vi "Waveform_Execution2.vi"(2 "output cluster":T1) -> ()   [LabVIEW 2013]
uses:
  waveforms.ctl
  <vilib>/DAQmx/create/channels.llb/DAQmx Create Channel (AO-Voltage-Basic).vi
  <vilib>/DAQmx/create/channels.llb/DAQmx Create Channel (DO-Digital Output).vi
  <vilib>/Waveform/WDTOps.llb/WDT Number of Waveform Samples DBL.vi
  <vilib>/DAQmx/configure/timing.llb/DAQmx Timing (Sample Clock).vi
  <vilib>/DAQmx/write.llb/DAQmx Write (Analog 1D Wfm NChan NSamp).vi
  <vilib>/DAQmx/configure/trigger.llb/DAQmx Start Trigger (Digital Edge).vi
  <vilib>/DAQmx/write.llb/DAQmx Write (Digital 1D Wfm NChan NSamp).vi
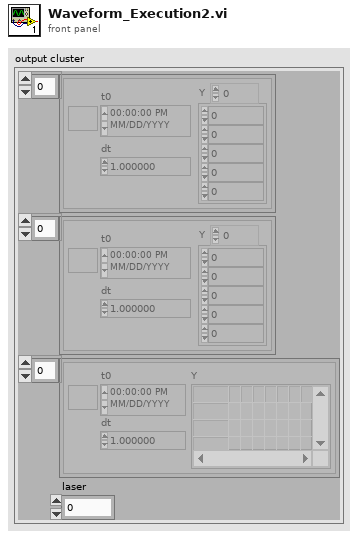
[diagram p1: front panel]
types:
  T1 = typedef "waveforms.ctl" = cluster{waveform(dbl)[], waveform(dbl)[], digitalwaveform[], "laser":i32}
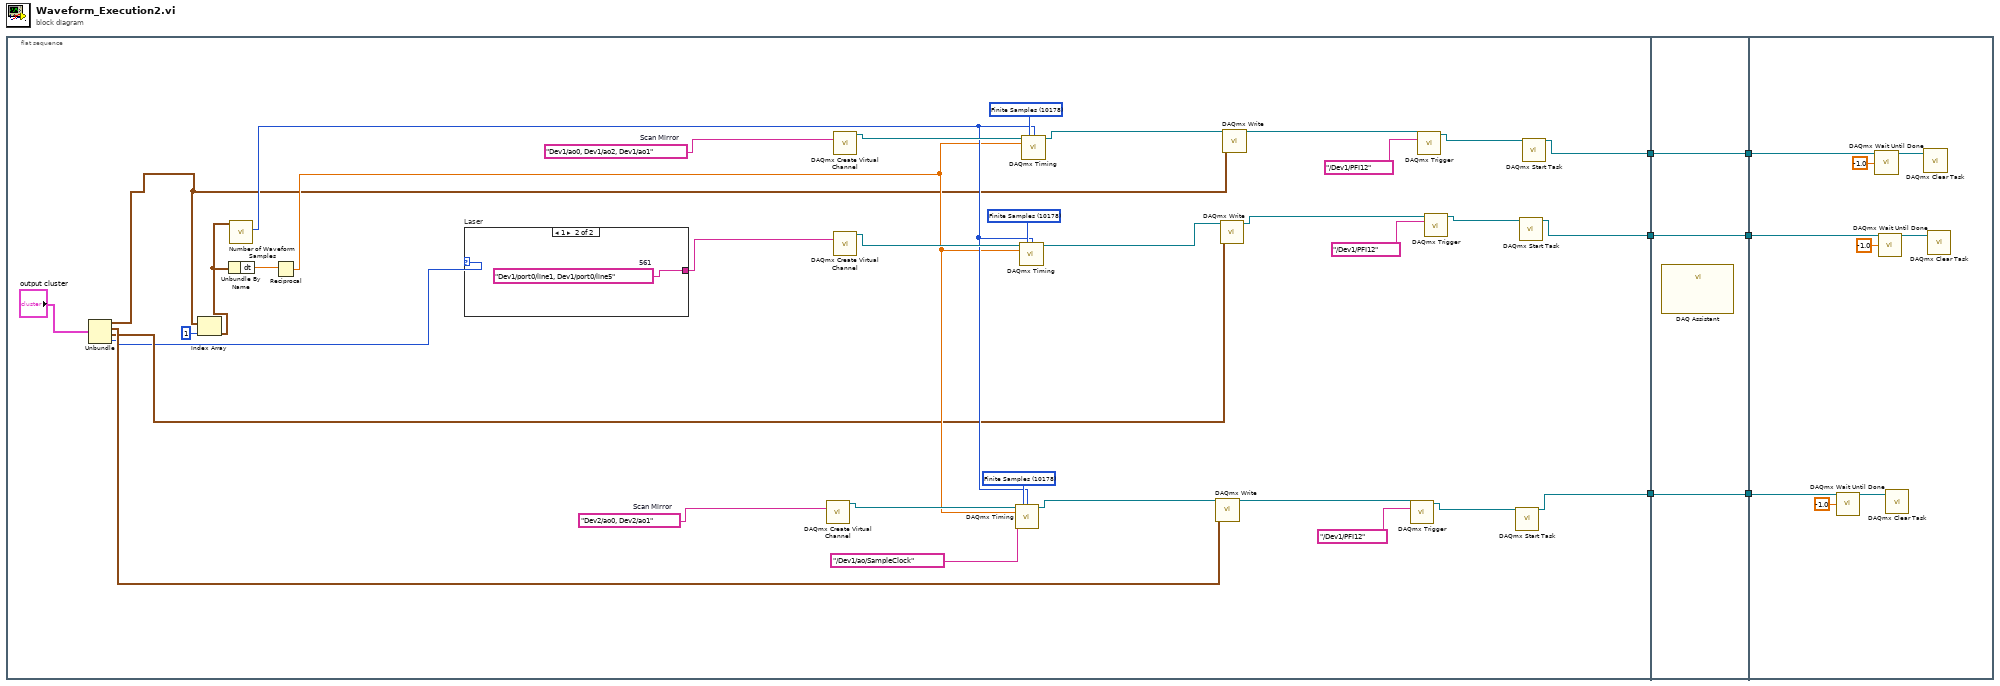
[diagram p0: block diagram]
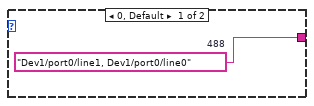
[diagram p2: hidden frame]
diagram:
  n1 = flat-sequence {
    tunnel: [w27] -> w5
    tunnel: [w26] -> w3
    tunnel: [w14] -> w1
    tunnel: [w46] -> w6
    tunnel: w5 -> [w46]
    tunnel: [w45] -> w4
    tunnel: w3 -> [w45]
    tunnel: [w44] -> w2
    tunnel: w1 -> [w44]
    tunnel: w6 -> [w53]
    tunnel: w4 -> [w52]
    tunnel: w2 -> [w47]
    frame #0 {
      w22 = 10178 items=["Finite Samples"=10178, "Continuous Samples"=10123, "Hardware Timed Single Point"=12522] ("sample mode")
      w23 = tag "Dev2/ao0, Dev2/ao1"  # Scan Mirror
      w39 = 10178 items=["Finite Samples"=10178, "Continuous Samples"=10123, "Hardware Timed Single Point"=12522] ("sample mode")
      w40 = 10178 items=["Finite Samples"=10178, "Continuous Samples"=10123, "Hardware Timed Single Point"=12522] ("sample mode")
      w41 = tag "Dev1/ao0, Dev1/ao2, Dev1/ao1"  # Scan Mirror
      n2 = Unbundle("output cluster") -> (w11:waveform(dbl)[], w10:waveform(dbl)[], w9:digitalwaveform[], "laser"=w8:i32)
      n3 = Index Array(array=w11, index=1) -> (element=w24:waveform(dbl))
      n4 = Unbundle By Name(w24) -> ("dt"=w34:dbl)
      n5 = call-poly <vilib>:"Number of Waveform Samples.vi"("waveform in"=w24) -> ("number of samples"=w16:i32)  [unwired: 8 in, 2 out]
      n6 = Reciprocal(x=w34) -> (1/x=w15:dbl)
      n7 = case "Laser" shown="1" w8 {
        tunnel: [w42 w43] -> w12
        frame 0, Default {
          w42 = tag "Dev1/port0/line1, Dev1/port0/line0"  # 488
        }
        frame 1 {
          w43 = tag "Dev1/port0/line1, Dev1/port0/line5"  # 561
        }
      }
      n8 = call-poly <vilib>:"DAQmx Create Virtual Channel.vi"("physical channels"=w23) -> ("task out"=w21:refnum<k21>)  [unwired: 13 in, 1 out]
      n9 = call-poly <vilib>:"DAQmx Create Virtual Channel.vi"("physical channels"=w41) -> ("task out"=w38:refnum<k21>)  [unwired: 13 in, 1 out]
      n10 = call-poly <vilib>:"DAQmx Create Virtual Channel.vi"("lines"=w12) -> ("task out"=w37:refnum<k21>)  [unwired: 13 in, 1 out]
      n11 = call-poly <vilib>:"DAQmx Timing.vi"("task/channels in"=w21, "sample mode"=w22, "samples per channel"=w16, "rate"=w15, "source"=tag "/Dev1/ao/SampleClock") -> ("task out"=w20:refnum<k21>)  [unwired: 9 in, 1 out]
      n12 = call-poly <vilib>:"DAQmx Timing.vi"("task/channels in"=w37, "sample mode"=w39, "samples per channel"=w16, "rate"=w15) -> ("task out"=w35:refnum<k21>)  [unwired: 10 in, 1 out]
      n13 = call-poly <vilib>:"DAQmx Timing.vi"("task/channels in"=w38, "sample mode"=w40, "samples per channel"=w16, "rate"=w15) -> ("task out"=w36:refnum<k21>)  [unwired: 10 in, 1 out]
      n14 = call-poly <vilib>:"DAQmx Write.vi"("task/channels in"=w20, "data"=w10) -> ("task out"=w18:refnum<k21>)  [unwired: 3 in, 10 out]
      n15 = call-poly <vilib>:"DAQmx Write.vi"("task/channels in"=w35, "data"=w9) -> ("task out"=w30:refnum<k21>)  [unwired: 3 in, 10 out]
      n16 = call-poly <vilib>:"DAQmx Write.vi"("task/channels in"=w36, "data"=w11) -> ("task out"=w31:refnum<k21>)  [unwired: 3 in, 10 out]
      n17 = call-poly <vilib>:"DAQmx Trigger.vi"("task/channels in"=w18, "source"=tag "/Dev1/PFI12") -> ("task out"=w17:refnum<k21>)  [unwired: 12 in, 1 out]
      n18 = call-poly <vilib>:"DAQmx Trigger.vi"("task/channels in"=w31, "source"=tag "/Dev1/PFI12") -> ("task out"=w29:refnum<k21>)  [unwired: 12 in, 1 out]
      n19 = call-poly <vilib>:"DAQmx Trigger.vi"("task/channels in"=w30, "source"=tag "/Dev1/PFI12") -> ("task out"=w28:refnum<k21>)  [unwired: 12 in, 1 out]
      n20 = call <vilib>:"DAQmx Start Task.vi"("task/channels in"=w17) -> ("task out"=w14:refnum<k21>)  [unwired: 1 in, 13 out]
      n21 = call <vilib>:"DAQmx Start Task.vi"("task/channels in"=w28) -> ("task out"=w26:refnum<k21>)  [unwired: 1 in, 13 out]
      n22 = call <vilib>:"DAQmx Start Task.vi"("task/channels in"=w29) -> ("task out"=w27:refnum<k21>)  [unwired: 1 in, 13 out]
    }
    frame #1 {
      n23 = call "DAQ Assistant"() -> ()  [unwired: 18 in, 2 out]
    }
    frame #2 {
      n24 = call <vilib>:"DAQmx Wait Until Done.vi"("task/channels in"=w47, "timeout (sec)"=-1.0) -> ("task out"=w49:refnum<k21>)  [unwired: 12 in, 1 out]
      n25 = call <vilib>:"DAQmx Wait Until Done.vi"("task/channels in"=w53, "timeout (sec)"=-1.0) -> ("task out"=w55:refnum<k21>)  [unwired: 12 in, 1 out]
      n26 = call <vilib>:"DAQmx Wait Until Done.vi"("task/channels in"=w52, "timeout (sec)"=-1.0) -> ("task out"=w54:refnum<k21>)  [unwired: 12 in, 1 out]
      n27 = call <vilib>:"DAQmx Clear Task.vi"("task in"=w49) -> ()  [unwired: 1 in, 14 out]
      n28 = call <vilib>:"DAQmx Clear Task.vi"("task in"=w55) -> ()  [unwired: 1 in, 14 out]
      n29 = call <vilib>:"DAQmx Clear Task.vi"("task in"=w54) -> ()  [unwired: 1 in, 14 out]
    }
  }
